vi "Compress.vi"(8 "Error In":errorcluster, 10 "StringData":string, 11 "reference in":refnum<class "CompressionDecorator.lvclass">) -> (0 "Error Out":errorcluster, 2 "Return(STRING)":string, 3 "reference in":refnum<class "CompressionDecorator.lvclass">)   [LabVIEW 2020, in "CompressionDecorator.lvclass"]
uses:
  CompressionDecorator.lvclass
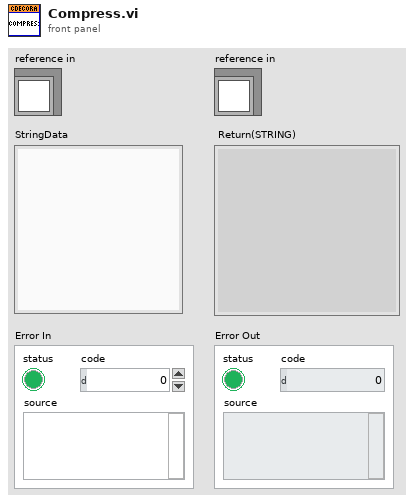
[diagram p1: front panel]
types:
  T1 = typedef "CompressionDecorator.lvclass/ObjectAttributes.ctl" = cluster{"CompLevel":i32}
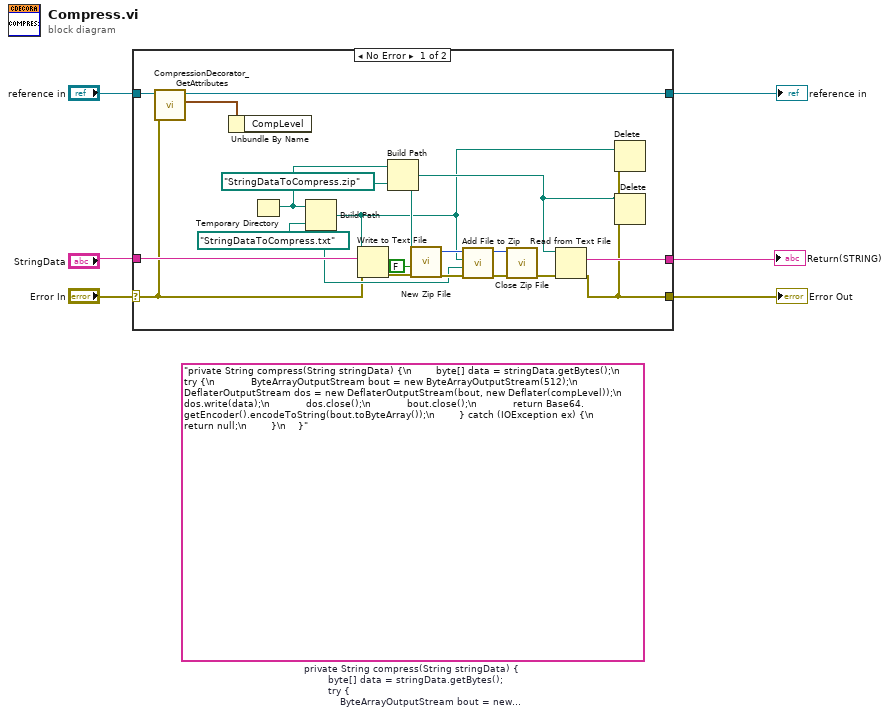
[diagram p0: block diagram]
diagram:
  (unwired) "private String compress(String stringData) {\n        byte[] data = stringData.getBytes();\n        try {\n            ByteArrayOutputStream bout = new ByteArrayOutputStream(512);\n            DeflaterOutputStream dos = new DeflaterOutputStream(bout, new Deflater(compLevel));\n            dos.write(data);\n            dos.close();\n            bout.close();\n            return Base64.getEncoder().encodeToString(bout.toByteArray());\n        } catch (IOException ex) {\n            return null;\n        }\n    }"  # private String compress(String stringData) {         byte[] data = stringData.getBytes();         try {             ByteArrayOutputStream bout = new ByteArrayOutputStream(512);             DeflaterOutputStream dos = new DeflaterOutputStream(bout, new Deflater(compLevel));             dos.write(data);             dos.close();             bout.close();             return Base64.getEncoder().encodeToString(bout.toByteArray());         } catch (IOException ex) {             return null;         }     }
  n1 = case shown="No Error" "Error In" {
    selector: "Error In" -> [w7 w27]
    tunnel: [w10 w27] -> w5
    tunnel: [w24 w26] -> w3
    tunnel: "reference in" -> [w25 w26]
    tunnel: "StringData" -> [w22 _]
    tunnel: [w12 _] -> w1
    frame No Error {
      w8 = path "StringDataToCompress.txt" ("name or relative path")
      n2 = call "CompressionDecorator_GetAttributes.vi"("error in (no error)"=w7, "reference in"=w25) -> ("Data"=w23:T1, "reference out"=w24:refnum<class "CompressionDecorator.lvclass">)  [unwired: 6 in, 2 out]
      n3 = Unbundle By Name(w23) -> ()  [unwired: 1 out]
      n4 = Temporary Directory() -> (w20:path)
      n5 = Build Path(base path=w20, name or relative path=w8) -> (appended path=w9:path)
      n6 = Write to Text File(file (use dialog)=w9, text=w22, error in=w7) -> (error out=w21:errorcluster)  [unwired: 1 in, 2 out]
      n7 = Build Path(base path=w20, name or relative path=path "StringDataToCompress.zip") -> (appended path=w11:path)
      n8 = call <vilib>:"New Zip File.vi"("error in (no error)"=w21, "confirm overwrite? (F)"=FALSE, "target"=w11) -> ("error out"=w17:errorcluster, "zip file out"=w16:i64)  [unwired: 2 in, 1 out]
      n9 = call <vilib>:"Add File to Zip.vi"("error in (no error)"=w17, "destination path in zip"=w8, "source file path"=w9, "zip file in"=w16) -> ("error out"=w15:errorcluster, "zip file out"=w14:i64)  [unwired: 6 in]
      n10 = call <vilib>:"Close Zip File.vi"("error in (no error)"=w15, "zip file in"=w14) -> ("error out"=w13:errorcluster)  [unwired: 5 in]
      n11 = Read from Text File(file (use dialog)=w11, error in=w13) -> (text=w12:string, error out=w10:errorcluster)  [unwired: 2 in, 2 out]
      n12 = Delete(path (use dialog)=w9, error in=w10) -> ()  [unwired: 3 in, 3 out]
      n13 = Delete(path (use dialog)=w11, error in=w10) -> ()  [unwired: 3 in, 3 out]
    }
    frame Error {
    }
  }
  "Error Out" <- w5
  "reference in" <- w3
  "Return(STRING)" <- w1
